vi "字符串转为浮点.vi"(1 "字符串":string) -> (0 "值":dbl)   [LabVIEW 2016]
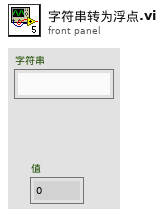
[diagram p1: front panel]
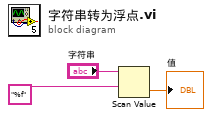
[diagram p0: block diagram]
diagram:
  n1 = Scan Value(string="字符串", format string="%f" ("格式字符串")) -> (value=→"值":dbl)  [unwired: 1 in, 1 out]
